vi "Qd Function Global.vi"(11 "Action":T1) -> (3 "Queued":u16)   [LabVIEW 2010, in "CAN Log Transfer and Convert.lvlib"]
uses:
  CAN Log Transfer and Convert.lvlib
  Qd Functional Global Action.ctl
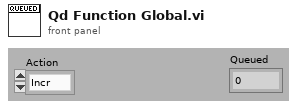
[diagram p1: front panel]
types:
  T1 = typedef "CAN Log Transfer and Convert.lvlib/Qd Functional Global Action.ctl" = enum16{"Incr", "Reset", "Get"}
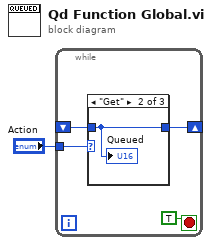
[diagram p0: block diagram]
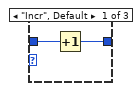
[diagram p2: hidden frame]
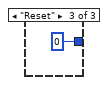
[diagram p3: hidden frame]
diagram:
  n1 = while {
    shift-right: [w4] -> _
    shift-left: _ -> [w3]
    tunnel: "Action" -> [w5]
    stop <- TRUE stop-if-true
    n2 = case shown="\"Get\"" w5 {
      tunnel: [w6 w8 u16 0] -> w4
      tunnel: w3 -> [w7 w8 _]
      frame "Incr", Default {
        n3 = Increment(x=w7) -> (x+1=w6:u16)
      }
      frame "Get" {
        "Queued" <- w8
      }
      frame "Reset" {
      }
    }
  }
